vi "Get PrimeTimer Q.vi"(8 "error in (no error)":errorcluster) -> (0 "error out":errorcluster, 1 "ElementData[]":variant[](array[variant]), 2 "ElementNames[]":string[](array[string]), 3 "DaqData ElapsedTimeRef":T1)   [LabVIEW 2022 SP3, in "DAQ.lvclass"]
doc: "Developed by Kevin Thompson\nThompson Engineering, LLC\nkevin@thompsonengineering.net"
uses:
  TD DaqLoopTime DataQ--ref.ctl
  GBL DataQ Refs.vi
  DAQ.lvclass
  DAQ.lvclass/DAQ.ctl
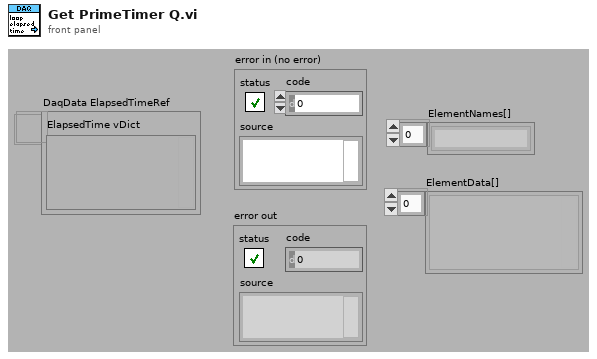
[diagram p1: front panel]
types:
  T1 = typedef "DAQ.lvclass/TD DaqLoopTime DataQ--ref.ctl" = refnum<queue>
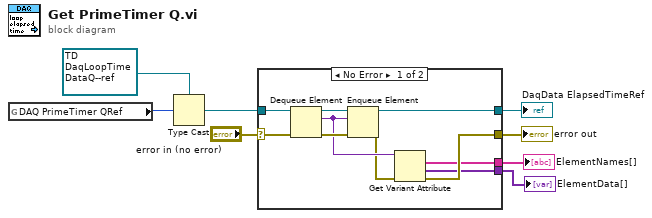
[diagram p0: block diagram]
diagram:
  n1 = global read "GBL DataQ Refs.vi" "DAQ PrimeTimer QRef"() -> (w5:u32)
  n2 = Type Cast(type=T1 refnum ("DaqData ElapsedTimeRef"), x=w5) -> (*(type *) &x=w4:T1)
  n3 = case shown="No Error" "error in (no error)" {
    selector: "error in (no error)" -> [w15 w19]
    tunnel: w4 -> [w16 w20]
    tunnel: [w12 w19] -> w8
    tunnel: [w14 w20] -> w7
    tunnel: [w11 _] -> w1
    tunnel: [w10 _] -> w2
    frame No Error {
      n4 = Dequeue Element(queue=w16, error in (no error)=w15) -> (queue out=w18:T1, element=w13:variant, error out=w17:errorcluster)  [unwired: 1 in, 1 out]
      n5 = Enqueue Element(queue=w18, element=w13, error in (no error)=w17) -> (queue out=w14:T1, error out=w9:errorcluster)  [unwired: 1 in, 1 out]
      n6 = Get Variant Attribute(Variant=w13, error in=w9) -> (names=w10:string[], values=w11:variant[], error out=w12:errorcluster)  [unwired: 2 in, 1 out]
    }
    frame Error {
    }
  }
  "DaqData ElapsedTimeRef" <- w7
  "error out" <- w8
  "ElementNames[]" <- w2
  "ElementData[]" <- w1
